vi "zmq_socket_set.vi"(3 "error in":errorcluster, 4 "socket":u64, 5 "context":u64) -> (0 "error out":errorcluster, 2 "socket out":refnum<class "zmq_socket.lvclass">)   [LabVIEW 2020, in "zeromq.lvlib" / "zmq_socket.lvclass"]
uses:
  zmq_socket.lvclass
  zmq_socket.lvclass/zmq_socket.ctl
panel:
  # "ØMQ"
  # "labview"
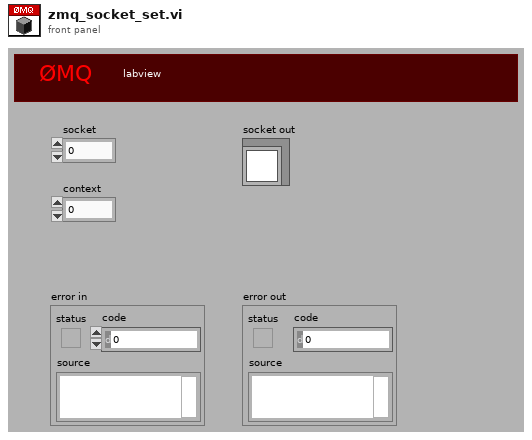
[diagram p1: front panel]
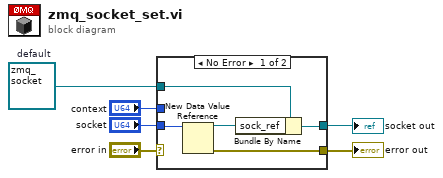
[diagram p0: block diagram]
diagram:
  w6 = refnum<class "zmq_socket.lvclass"> refnum  # default
  n1 = case shown="No Error" "error in" {
    selector: "error in" -> [_ w12]
    tunnel: w6 -> [w11 _]
    tunnel: [w10 _] -> w5
    tunnel: [w7 w12] -> w3
    tunnel: "context" -> [_ _]
    tunnel: "socket" -> [w8 _]
    frame No Error {
      n2 = New Data Value Reference(data value=w8) -> (data value reference=w9:refnum<data-value>, error out=w7:errorcluster)  [unwired: 1 in]
      n3 = Bundle By Name(cluster=w11, "sock_ref"=w9) -> (w10:refnum<class "zmq_socket.lvclass">)
    }
    frame Error {
    }
  }
  "socket out" <- w5
  "error out" <- w3
